vi "Duplicate_DO_WF.vi"(8 "error in":errorcluster) -> (0 "error out":errorcluster)   [LabVIEW 2025]
uses:
  <vilib>/Waveform/DWDTOps.llb/DWDT Append Digital Samples.vi
  <vilib>/Waveform/DWDTOps.llb/DWDT Digital Size.vi
panel:
  out "Digital waveform 3":digitalwaveform[](graph)
  out "Samples":u32
  in  "Digital waveform 2":digitalwaveform[](graph)
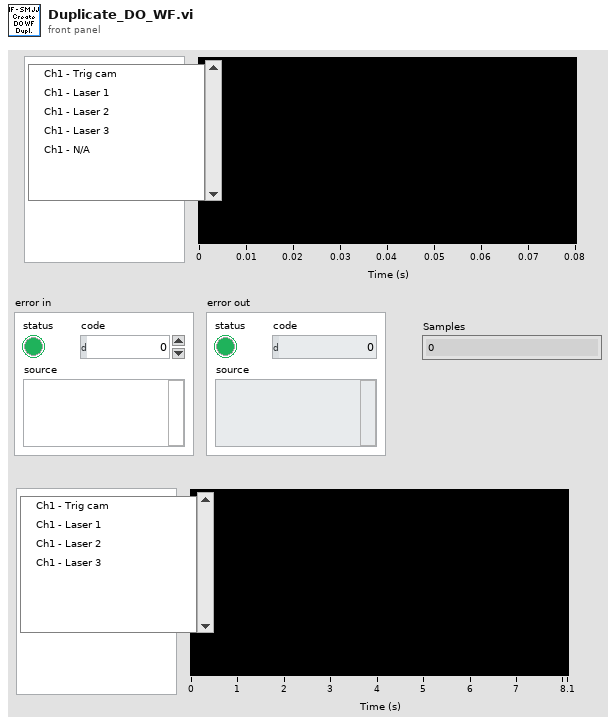
[diagram p1: front panel]
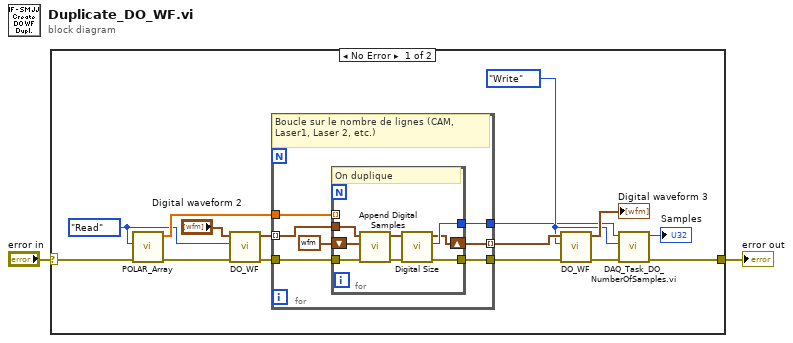
[diagram p0: block diagram]
diagram:
  n1 = case shown="No Error" "error in" {
    selector: "error in" -> [w12 w33]
    tunnel: [w3 w33] -> w1
    frame No Error {
      w9 = enum16{"Write", "Read"}."Read" ("Action")
      w7 = enum16{"Write", "Read"}."Write" ("Action")
      n2 = call "POLAR_Array.vi"("error in"=w12, "Action"=w9) -> ("error out"=w11:errorcluster, "Pockels_Array"=w10:dbl[])  [unwired: 8 in]
      n3 = call "DO_WF.vi"("error in"=w11, "Action"=w9, "Digital WF"="Digital waveform 2") -> ("error out"=w16:errorcluster, "Digital WF"=w15:digitalwaveform[])  [unwired: 7 in]
      n4 = for {
        tunnel: w15 -> [w24] mode=indexing
        tunnel: [w19] -> w8 mode=indexing
        tunnel: w10 -> [w22]
        tunnel: [w18] -> w6
        tunnel: w16 -> [w21]
        tunnel: [w20] -> w14
        # "Boucle sur le nombre de lignes (CAM, Laser1, Laser 2, etc.)"
        n5 = for {
          tunnel: w24 -> [w32]
          shift-right: [w25] -> w19
          shift-left: digitalwaveform {"t0"=timestamp(0 s since 1904-01-01), "dt"=1e-05, "Y"={"transitions"=[], "data"=[]}} ("digital waveform out") -> [w30]
          tunnel: w22 -> [_] mode=indexing
          tunnel: [w28] -> w18
          tunnel: w21 -> [w29]
          tunnel: [w26] -> w20
          # "On duplique"
          n6 = call-poly <vilib>:"Append Digital Samples.vi"("error in (no error)"=w29, "digital waveform B"=w30, "digital waveform A"=w32) -> ("error out"=w27:errorcluster, "digital waveform out"=w31:digitalwaveform)  [unwired: 7 in]
          n7 = call-poly <vilib>:"Digital Size.vi"("error in (no error)"=w27, "digital waveform in"=w31) -> ("error out"=w26:errorcluster, "number of samples"=w28:i32, "digital waveform out"=w25:digitalwaveform)  [unwired: 6 in, 1 out]
        }
      }
      n8 = call "DO_WF.vi"("error in"=w14, "Action"=w7, "Digital WF"=w8) -> ("error out"=w5:errorcluster, "Digital WF"=→"Digital waveform 3":digitalwaveform[])  [unwired: 7 in]
      n9 = call "DAQ_Task_DO_NumberOfSamples.vi.vi"("error in"=w5, "Action"=w7, "Samples"=w6) -> ("error out"=w3:errorcluster, "Samples"=→"Samples":u32)  [unwired: 7 in]
    }
    frame Error {
    }
  }
  "error out" <- w1
